vi "SaveData.vi"(0 "object in":refnum<class "TDMSLogger_PowerScan.lvclass">, 1 "Elapsed Time":dbl, 2 "ChannelsWFIn":waveform(dbl)[](array[waveform]), 3 "AmplitudeAndVoltageSettings":T4, 4 "MeTecData":T3={"meTEC_CH2_Temperature Stability"=1, "meTEC_CH2_Act. Output Current [A]"=0.0, "meTEC_CH2_Act. Output Voltage [V]"=0.0, "meTEC_CH2_Object Temperature [°C]"=0.0, "meTEC_CH2_Sink Temperature [°C]"=0.0, "meTEC_CH1_Error Parameter"=0, "meTEC_CH1_Error Instance"=0, "meTEC_CH1_Error No."=0, "meTEC_CH1_Device Status"=1, "meTEC_CH1_Temperature Stability"=1, "meTEC_CH1_Act. Output Current [A]"=0.0, "meTEC_CH1_Act. Output Voltage [V]"=0.0, "meTEC_CH1_Object Temperature [°C]"=0.0, "meTEC_CH1_Sink Temperature [°C]"=0.0} {"meTEC_CH1_Sink Temperature [°C]" format="%.3f"; "meTEC_CH1_Object Temperature [°C]" format="%.3f"; "meTEC_CH1_Act. Output Voltage [V]" format="%.3f"; "meTEC_CH1_Act. Output Current [A]" format="%.3f"; "meTEC_CH1_Temperature Stability" items=["Temperature regulation is not active", "Is not stable", "Is stable"]; "meTEC_CH1_Device Status" items=["Initializing", "Ready", "Run", "Error", "Bootloader", "Reset in Progress"]; "meTEC_CH2_Sink Temperature [°C]" format="%.3f"; "meTEC_CH2_Object Temperature [°C]" format="%.3f"; "meTEC_CH2_Act. Output Voltage [V]" format="%.3f"; "meTEC_CH2_Act. Output Current [A]" format="%.3f"; "meTEC_CH2_Temperature Stability" items=["Temperature regulation is not active", "Is not stable", "Is stable"]}, 5 "error in (no error)":errorcluster, 6 "AGTemp":dbl, 7 "SetPower":dbl, 8 "MCCTempdata":dbl[](array[numeric]), 9 "MeasuredPower":dbl, 11 "AmplitudeOk":bool, 13 "WfgEnabled":cluster{"Ch1":bool, "Ch2":bool}) -> (14 "object out":refnum<class "TDMSLogger_PowerScan.lvclass">, 19 "error out":errorcluster)   [LabVIEW 2023, in "TDMSLogger_PowerScan.lvclass"]
uses:
  TDMSLogger_PowerScan.lvclass
  TDMSLogger_PowerScan.lvclass/TDMSLogger_PowerScan.ctl
  TEC LabVIEW Control Software v0.14/Source/LV Source/[meerstetter engineering TE Cooling]/TypeDefs/meTEC_ID 1200_Temperature is Stable.ctl
  TEC LabVIEW Control Software v0.14/Source/LV Source/[meerstetter engineering TE Cooling]/TypeDefs/meTEC_ID 104_Device Status.ctl
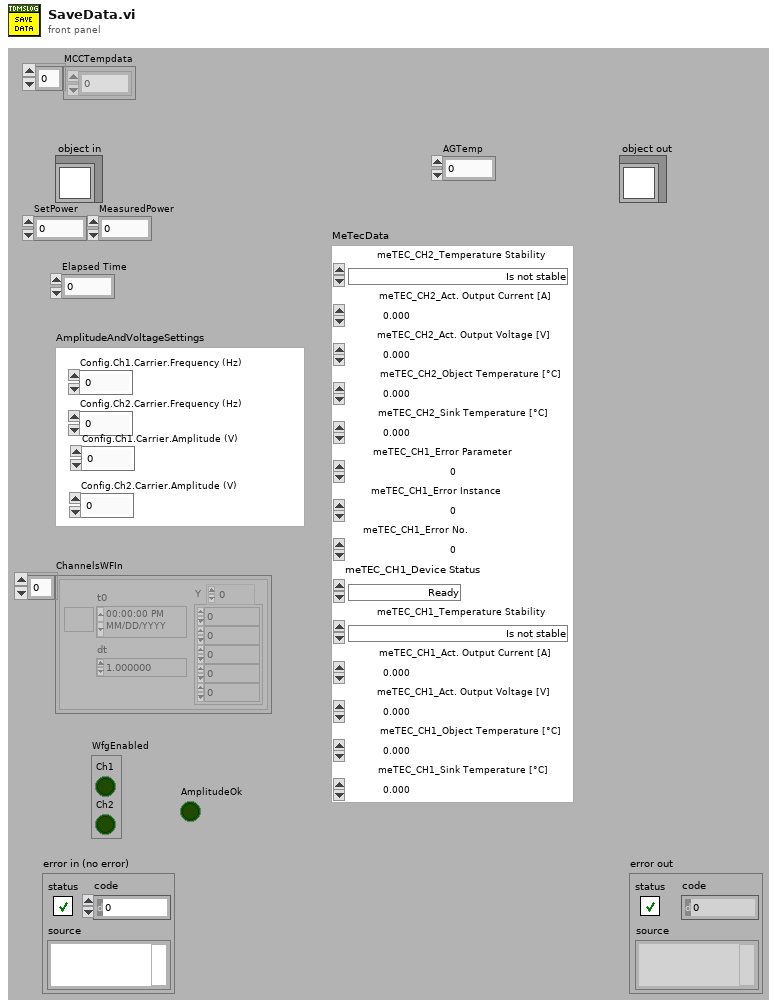
[diagram p1: front panel]
types:
  T1 = typedef "meTEC_ID 1200_Temperature is Stable.ctl" = i32
  T2 = typedef "meTEC_ID 104_Device Status.ctl" = i32
  T3 = cluster{"meTEC_CH2_Temperature Stability":T1, "meTEC_CH2_Act. Output Current [A]":dbl, "meTEC_CH2_Act. Output Voltage [V]":dbl, "meTEC_CH2_Object Temperature [°C]":dbl, "meTEC_CH2_Sink Temperature [°C]":dbl, "meTEC_CH1_Error Parameter":i32, "meTEC_CH1_Error Instance":i32, "meTEC_CH1_Error No.":i32, "meTEC_CH1_Device Status":T2, "meTEC_CH1_Temperature Stability":T1, "meTEC_CH1_Act. Output Current [A]":dbl, "meTEC_CH1_Act. Output Voltage [V]":dbl, "meTEC_CH1_Object Temperature [°C]":dbl, "meTEC_CH1_Sink Temperature [°C]":dbl}
  T4 = cluster{"Config.Ch1.Carrier.Frequency (Hz)":dbl, "Config.Ch2.Carrier.Frequency (Hz)":dbl, "Config.Ch1.Carrier.Amplitude (V)":dbl, "Config.Ch2.Carrier.Amplitude (V)":dbl}
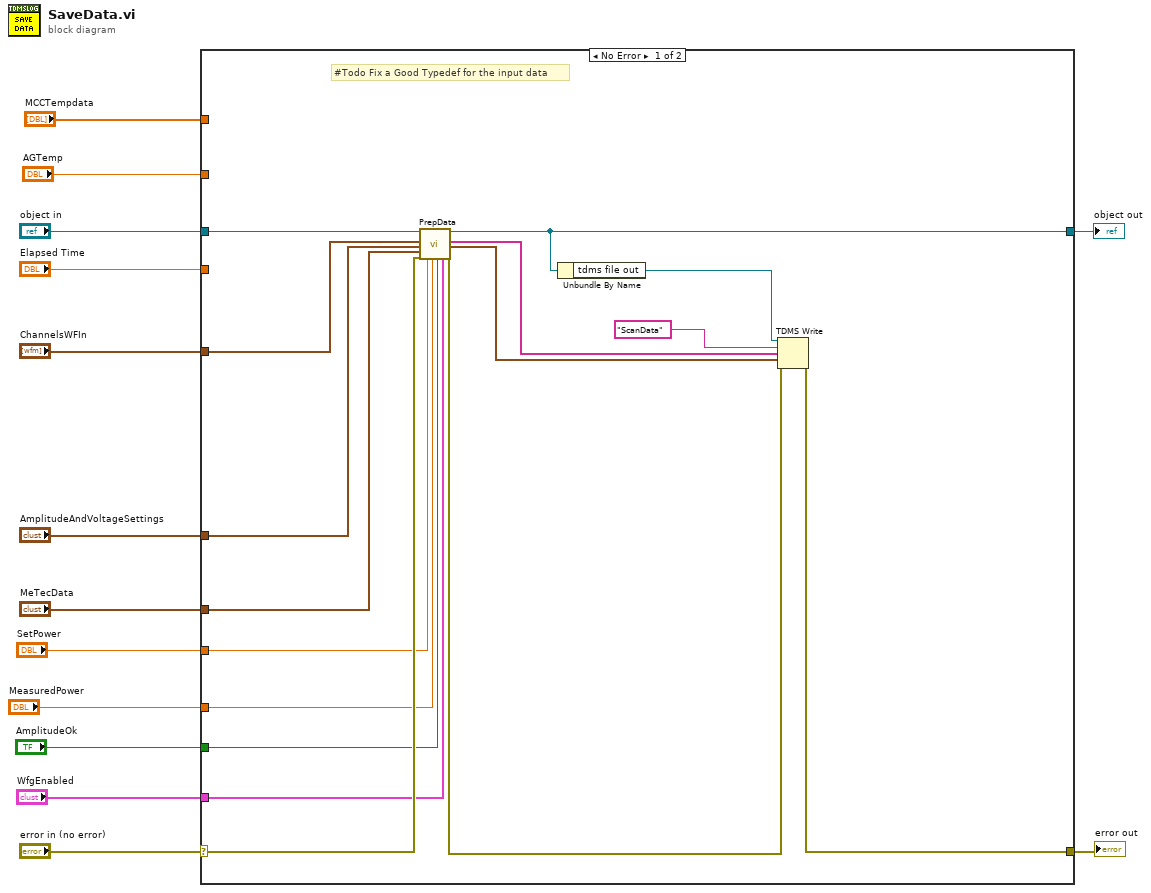
[diagram p0: block diagram]
diagram:
  n1 = case shown="No Error" "error in (no error)" {
    selector: "error in (no error)" -> [w24 w32]
    tunnel: [w27 w32] -> w13
    tunnel: [w22 w31] -> w11
    tunnel: "object in" -> [w26 w31]
    tunnel: "AmplitudeAndVoltageSettings" -> [w30 _]
    tunnel: "ChannelsWFIn" -> [w28 _]
    tunnel: "Elapsed Time" -> [_ _]
    tunnel: "MeTecData" -> [w25 _]
    tunnel: "SetPower" -> [w18 _]
    tunnel: "MeasuredPower" -> [w17 _]
    tunnel: "AmplitudeOk" -> [w16 _]
    tunnel: "WfgEnabled" -> [w15 _]
    tunnel: "AGTemp" -> [_ _]
    tunnel: "MCCTempdata" -> [_ _]
    frame No Error {
      # "#Todo Fix a Good Typedef for the input data"
      n2 = call-dynamic "PrepData.vi"("object in"=w26, "ChannelsWFIn"=w28, "AmplitudeAndVoltageSettings"=w30, "MeTecData"=w25, "error in (no error)"=w24, "SetPower"=w18, "MeasuredPower"=w17, "AmplitudeOk"=w16, "WfgEnabled"=w15) -> ("object out"=w22:refnum<class "TDMSLogger_PowerScan.lvclass">, "Channel Names"=w21:string[], "Channels(WF)"=w20:waveform(dbl)[], "error out"=w23:errorcluster)  [unwired: 7 in]
      n3 = Unbundle By Name(w22) -> ("tdms file out"=w19:refnum<k34>)
      n4 = TDMS Write(0:w19, 5:"ScanData" ("group name in (Untitled)"), 7:w21, 9:w20, 11:w23) -> (15:w27:errorcluster)  [unwired: 1 in, 3 out]
    }
    frame Error {
    }
  }
  "error out" <- w13
  "object out" <- w11
